vi "Main.vi"() -> ()   [LabVIEW 2017]
doc: "The myRIO Project template acquires acceleration data from the onboard accelerometer and displays the changes of acceleration values in a waveform chart."
uses:
  <vilib>/myRIO/Common/Instrument Driver Framework/myRIO v1.0/UART/vis/myRIO v1.0 Close UART.vi
  <vilib>/myRIO/Common/Instrument Driver Framework/Utilities/vis/FPGA Ref Manager.vi
  <vilib>/myRIO/Common/Instrument Driver Framework/myRIO v1.0/myRIO v1.0 Reset FPGA.vi
  <vilib>/myRIO/Common/Instrument Driver Framework/myRIO v1.0/IRQ/vis/myRIO v1.0 IRQ Info FGV.vi
  <vilib>/myRIO/Common/Instrument Driver Framework/myRIO v1.0/IRQ/vis/myRIO v1.0 Timer IRQ Info FGV.vi
  <vilib>/myRIO/Common/Instrument Driver Framework/myRIO v1.0/IRQ/vis/myRIO v1.0 ISR Agent.vi
  <vilib>/myRIO/Instrument Drivers/Utilities/Utilities.lvlib
panel:
  in  "I2C Configuration":T1
  out "Temp deg C":dbl
  out "error out":errorcluster
  in  "Stop":bool
  # "Overview: The myRIO Project template acquires acceleration data from the onboard accelerometer and displays the changes of acceleration values in a waveform chart.\nInstructions:\n1. Check the myRIO target IP address in the project and make sure the target IP address is correct. \n2. Run this VI."
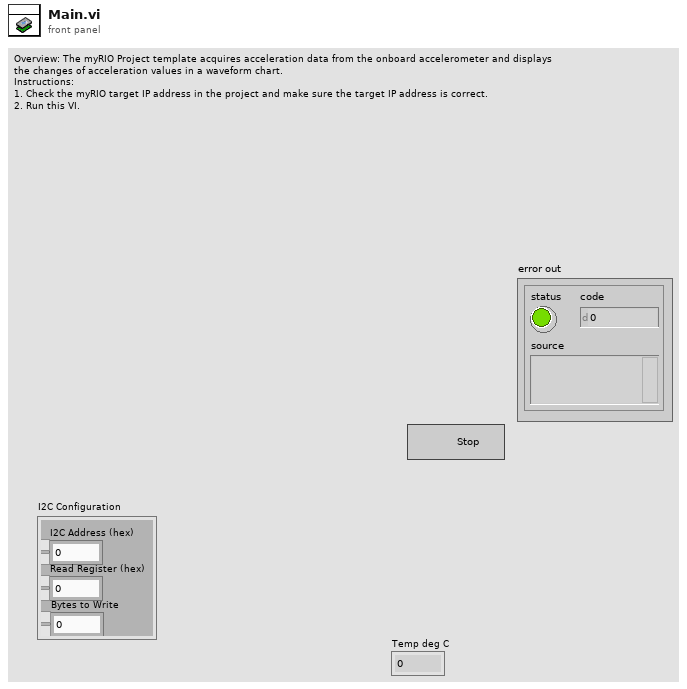
[diagram p1: front panel]
types:
  T1 = cluster{"I2C Address (hex)":dbl, "Read Register (hex)":dbl, "Bytes to Write":dbl}
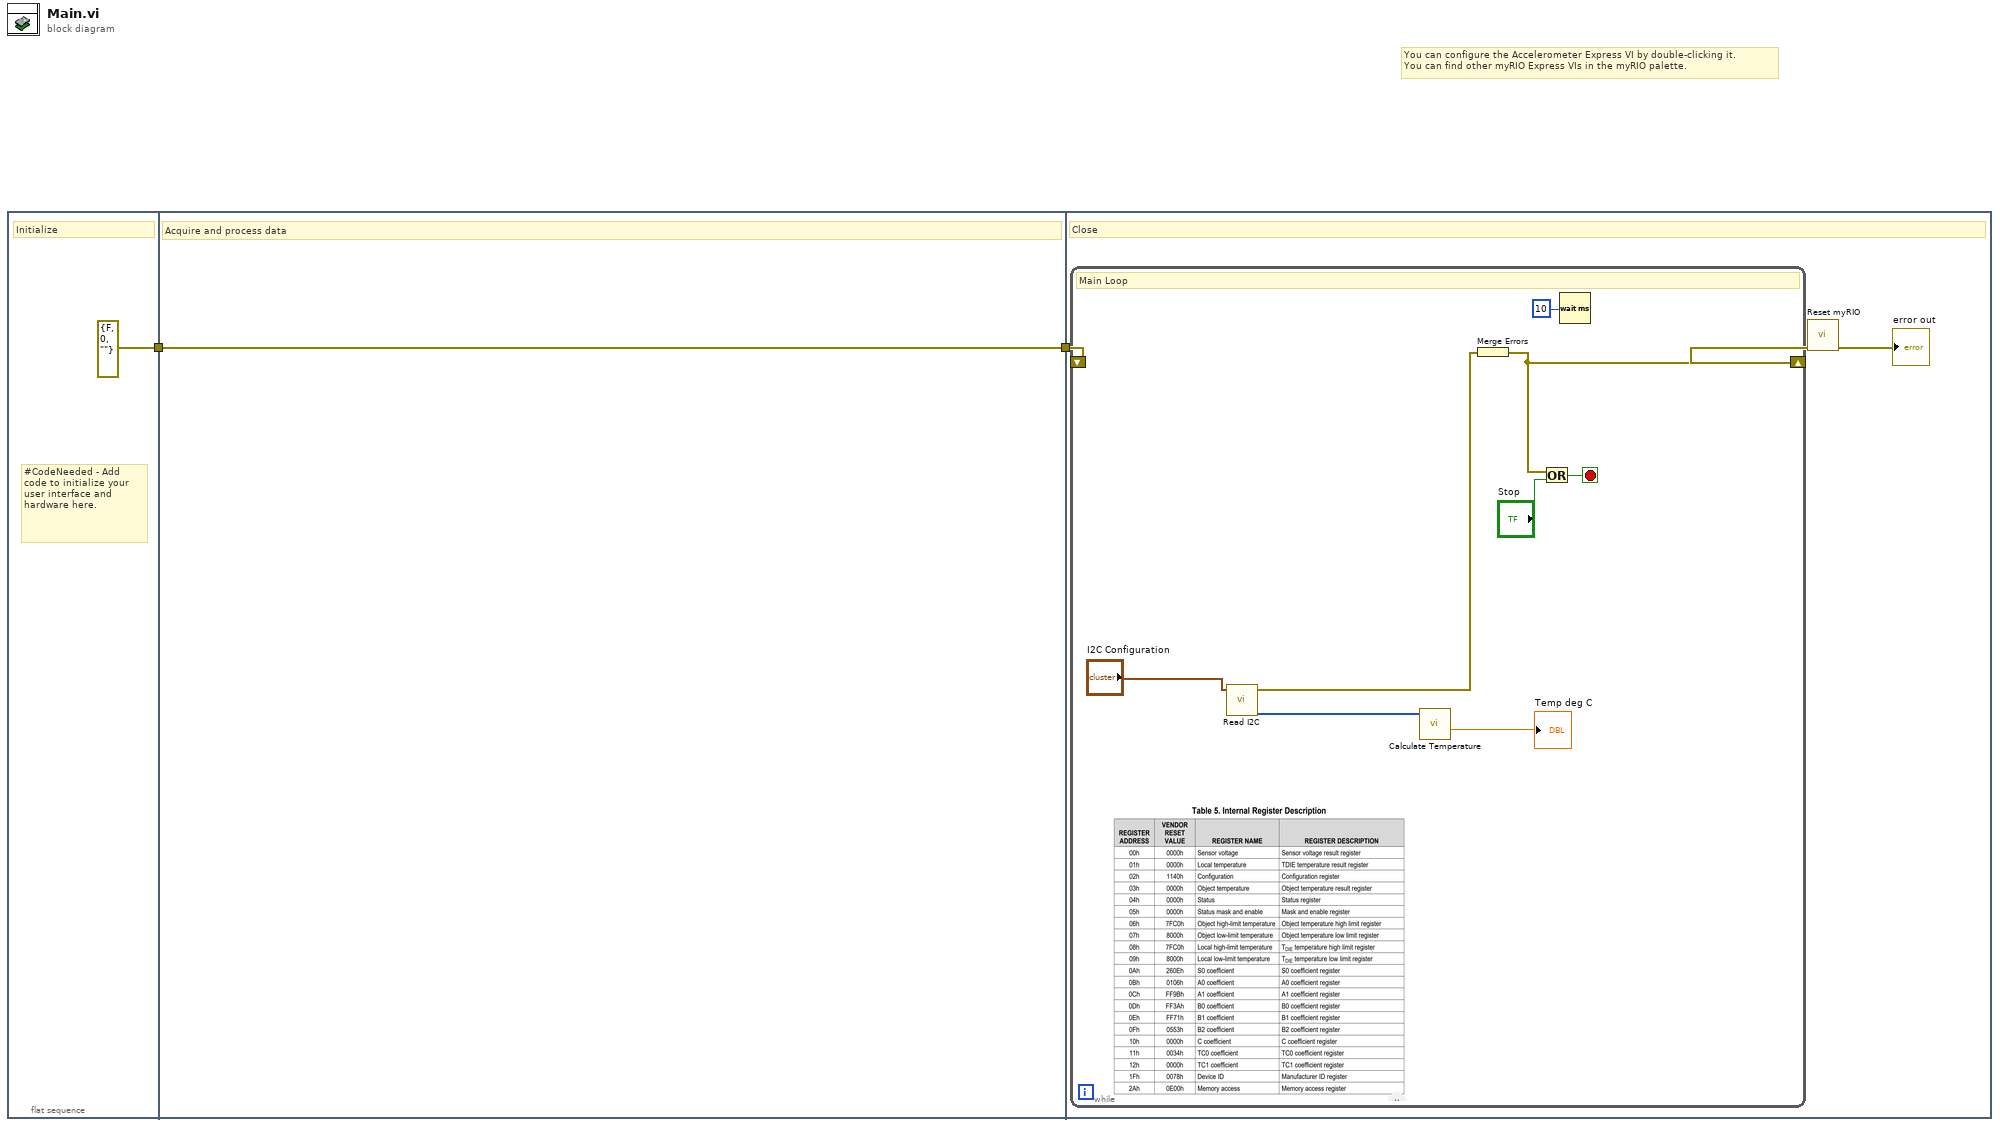
[diagram p0: block diagram]
diagram:
  # "You can configure the Accelerometer Express VI by double-clicking it.\nYou can find other myRIO Express VIs in the myRIO palette."
  n1 = flat-sequence {
    tunnel: [errorcluster {"status"=FALSE, "code"=0, "source"=""} ("error in (no error)")] -> w2
    tunnel: w2 -> [w4]
    tunnel: [w4] -> w1
    tunnel: w1 -> [w6]
    frame #0 {
      # "#CodeNeeded - Add code to initialize your user interface and hardware here."
      # "Initialize"
    }
    frame #1 {
      # "Acquire and process data"
    }
    frame #2 {
      # "Close"
      n2 = while {
        shift-right: [w12] -> w5
        shift-left: w6 -> [_]
        stop <- w14 stop-if-true
        # "Main Loop"
        n3 = call "Read I2C.vi"("I2C Channel Config"="I2C Configuration") -> ("Bytes Read"=w10:u8[], "error out"=w9:errorcluster)  [unwired: 9 in]
        n4 = call "Calculate Temperature.vi"("Bytes Read"=w10) -> ("Temp Deg C"=→"Temp deg C":dbl)  [unwired: 10 in]
        n5 = Merge Errors(w9) -> (w12:errorcluster)
        n6 = Or(x=w12, y="Stop") -> (x .or. y?=w14:bool)
        n7 = Wait (ms)(milliseconds to wait=u32 10) -> ()  [unwired: 1 out]
      }
      n8 = call <vilib>:"Reset myRIO.vi"("error in (no error)"=w5) -> ("error out"=→"error out":errorcluster)  [unwired: 10 in]
    }
  }
